vi "multi_plots_2d_data.vi"() -> ()   [LabVIEW 2022 SP3]
panel:
  out "Waveform Graph":dbl[][](graph)
  out "Waveform Chart":dbl[][](graph)
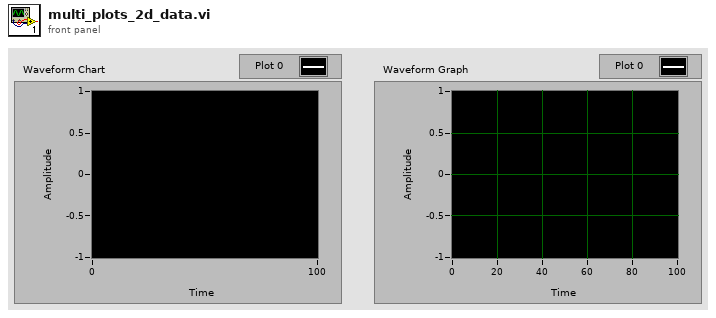
[diagram p1: front panel]
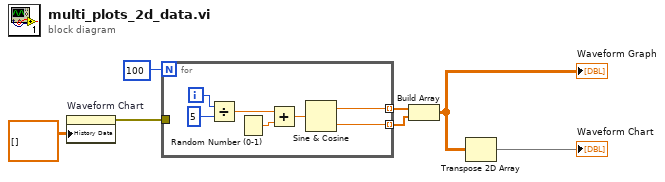
[diagram p0: block diagram]
diagram:
  n1 = property on="Waveform Chart" class="WFChart (严格)"("History Data"=dbl[][] []) -> (error out=w6:errorcluster)  [unwired: 2 in, 1 out]
  n2 = for {
    N: 100 -> [_]
    tunnel: [w9] -> w5 mode=indexing
    tunnel: w6 -> [_]
    tunnel: [w8] -> w3 mode=indexing
    i -> [w14]
    n3 = Divide(x=w14, y=5) -> (x/y=w11:dbl)
    n4 = Random Number (0-1)() -> (number: 0 to 1=w12:dbl)
    n5 = Add(x=w11, y=w12) -> (x+y=w10:dbl)
    n6 = Sine & Cosine(0:w10) -> (1:w9:dbl, 2:w8:dbl)
  }
  n7 = Build Array(w5, w3) -> (w2:dbl[][])
  "Waveform Graph" <- w2
  n8 = Transpose 2D Array(2D array=w2) -> (transposed array=→"Waveform Chart":dbl[][])
